vi "clearLicker.vi"(8 "error in (no error)":errorcluster, 11 "Licker in":refnum<class "Licker.lvclass">) -> (0 "error out":errorcluster, 3 "Licker out":refnum<class "Licker.lvclass">)   [LabVIEW 2014, in "Licker.lvclass"]
uses:
  Licker.lvclass
  Licker.lvclass/Licker.ctl
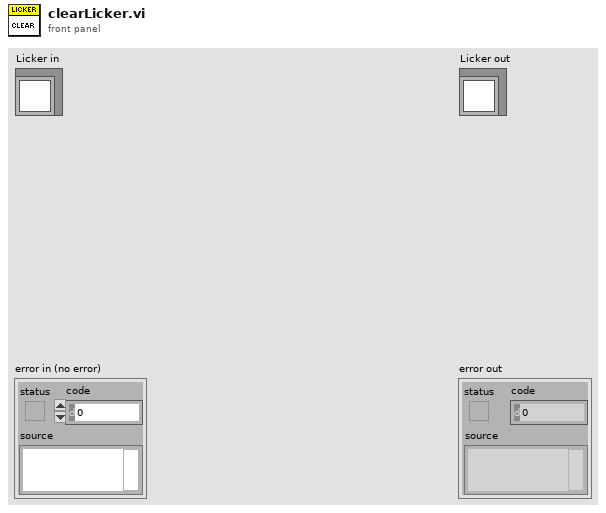
[diagram p1: front panel]
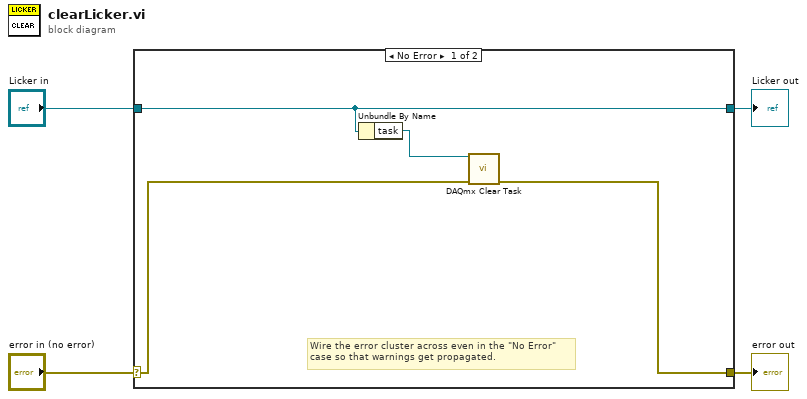
[diagram p0: block diagram]
diagram:
  n1 = case shown="No Error" "error in (no error)" {
    selector: "error in (no error)" -> [w6 w10]
    tunnel: [w5 w10] -> w3
    tunnel: [w8 w9] -> w1
    tunnel: "Licker in" -> [w8 w9]
    frame No Error {
      # "Wire the error cluster across even in the \"No Error\"\ncase so that warnings get propagated."
      n2 = Unbundle By Name(w8) -> ("task"=w7:refnum<k21>)
      n3 = call <vilib>:"DAQmx Clear Task.vi"("task in"=w7, "error in"=w6) -> ("error out"=w5:errorcluster)  [unwired: 13 in]
    }
    frame Error {
    }
  }
  "error out" <- w3
  "Licker out" <- w1
